vi "LoadResultsFromFile.vi"(8 "error in (no error)":errorcluster, 11 "ResultsViewer in":refnum<class "ResultsViewer.lvclass">) -> (0 "error out":errorcluster, 3 "ResultsViewer out":refnum<class "ResultsViewer.lvclass">)   [LabVIEW 2019, in "ResultsViewer.lvlib" / "ResultsViewer.lvclass"]
uses:
  ResultsViewer.lvclass
  ResultsViewer.lvclass/ResultsViewer.ctl
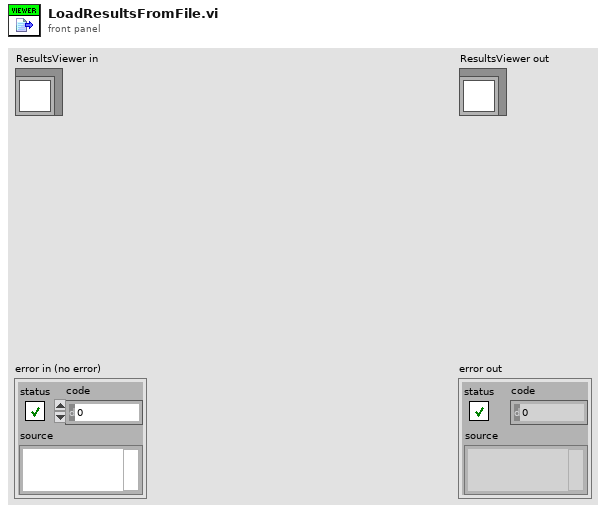
[diagram p1: front panel]
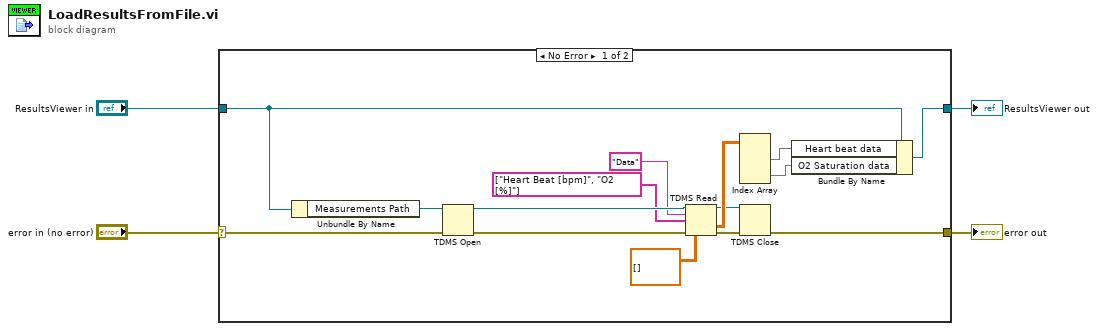
[diagram p0: block diagram]
diagram:
  n1 = case shown="No Error" "error in (no error)" {
    selector: "error in (no error)" -> [w8 w21]
    tunnel: [w7 w21] -> w3
    tunnel: [w18 w20] -> w1
    tunnel: "ResultsViewer in" -> [w19 w20]
    frame No Error {
      n2 = Unbundle By Name(w19) -> ("Measurements Path"=w9:path)
      n3 = TDMS Open(8:w8, 11:w9) -> (0:w14:errorcluster, 3:w13:refnum<k34>)  [unwired: 5 in]
      n4 = TDMS Read(0:w13, 5:"Data" ("group name in (Untitled)"), 7:string[] ["Heart Beat [bpm]", "O2 [%]"] ("channel name(s) in (Untitled)"), 11:w14, 12:dbl[][] []) -> (4:w15:refnum<k34>, 10:w17:dbl[][], 15:w16:errorcluster)  [unwired: 3 in, 3 out]
      n5 = Index Array(array=w17) -> (element #1=w6:dbl[], element #2=w5:dbl[])  [unwired: 4 in]
      n6 = TDMS Close(8:w16, 11:w15) -> (0:w7:errorcluster)  [unwired: 1 out]
      n7 = Bundle By Name(cluster=w19, "Heart beat data"=w6, "O2 Saturation data"=w5) -> (w18:refnum<class "ResultsViewer.lvclass">)
    }
    frame Error {
    }
  }
  "error out" <- w3
  "ResultsViewer out" <- w1
